vi "SetTC_K.vi"(8 "error in":errorcluster, 11 "CN79000 in":refnum<class "CN79000.lvclass">) -> (0 "error out":errorcluster, 3 "CN79000 out":refnum<class "CN79000.lvclass">)   [LabVIEW 2012, in "CN79000.lvclass"]
uses:
  CN79000.lvclass
  Build Command-Single Val.vi
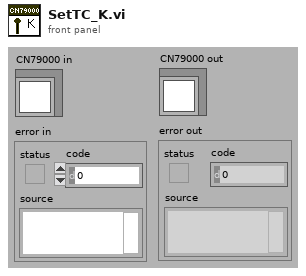
[diagram p1: front panel]
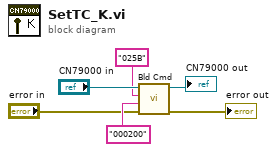
[diagram p0: block diagram]
diagram:
  n1 = call-poly "Bld Cmd.vi"("error in"="error in", "Val"="000200" ("Cmd"), "Cmd"="025B" ("string"), "CN79000 in"="CN79000 in") -> ("error out"=→"error out":errorcluster, "CN79000 out"=→"CN79000 out":refnum<class "CN79000.lvclass">)  [unwired: 3 in, 2 out]
